vi "Query Assets.vi"(8 "Error In":errorcluster, 10 "Asset Filter":string, 11 "Session In":refnum<class "NI Skyline Configuration HTTP.lvclass">) -> (0 "Error Out":errorcluster, 2 "Assets":T1(array[cluster]), 3 "Session Out":refnum<class "NI Skyline Configuration HTTP.lvclass">)   [LabVIEW 2019]
uses:
  <vilib>/Skyline/Configuration/Configuration HTTP_class/NI Skyline Configuration HTTP.lvclass
  <vilib>/httpClient/LabVIEWHTTPClient.lvlib
  <vilib>/httpClient/POSTBuffer.vi
panel:
  out "Server URL":string
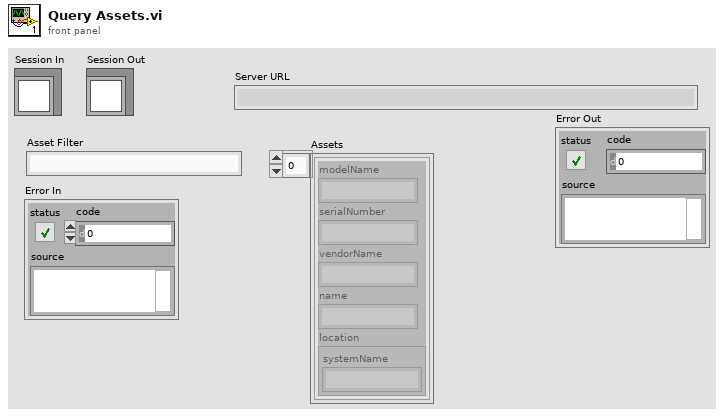
[diagram p1: front panel]
types:
  T1 = cluster{"modelName":string, "serialNumber":string, "vendorName":string, "name":string, "location":cluster{"systemName":string}}[]
  T2 = cluster{"modelName":string, "serialNumber":string, "vendorName":string, "name":string, "location":cluster{"systemName":string}}
  T3 = typedef "LabVIEWHTTPClient.lvlib/ClientHandle.ctl" = refnum<k1>
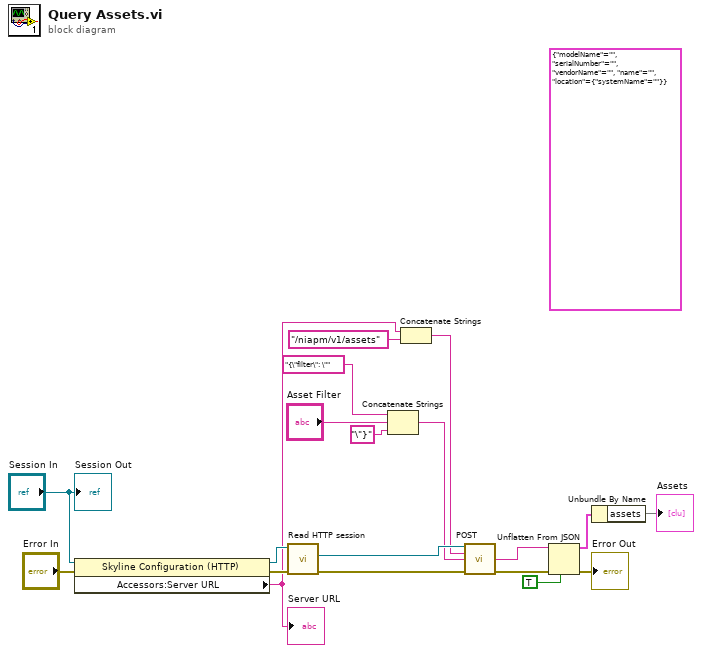
[diagram p0: block diagram]
diagram:
  (unwired) T2 {"modelName"="", "serialNumber"="", "vendorName"="", "name"="", "location"={"systemName"=""}} ("asset")
  n1 = property class="Skyline Configuration (HTTP)"(reference="Session In", error in="Error In") -> (reference out=w19:refnum<class "NI Skyline Configuration HTTP.lvclass">, error out=w18:errorcluster, "Accessors:Server URL"=w16:string)
  "Server URL" <- w16
  n2 = call <vilib>:"Read HTTP session.vi"("error in (no error)"=w18, "HTTP configuration in"=w19) -> ("error out"=w17:errorcluster, "http session"=w20:T3)  [unwired: 7 in, 1 out]
  n3 = Concatenate Strings("{\"filter\": \"" ("buffer"), "Asset Filter", "\"}" ("buffer")) -> (w11:string)
  n4 = Concatenate Strings(w16, "/niapm/v1/assets" ("string")) -> (w15:string)
  n5 = call-poly <vilib>:"POST.vi"("client handle"=w20, "url"=w15, "buffer"=w11, "error in (no error)"=w17) -> ("body"=w10:string, "error out"=w4:errorcluster)  [unwired: 8 in, 2 out]
  n6 = Unflatten From JSON(JSON string=w10, default null elements? (F)=TRUE, error in (no error)=w4) -> (type and defaults=w9:cluster{}, value=w2:cluster{}, error out=→"Error Out":errorcluster)  [unwired: 3 in]
  n7 = Unbundle By Name(w2) -> ("assets"=→"Assets")
  "Session Out" <- "Session In"
